vi "New Client Handle.vi"(8 "error in (no error)":errorcluster, 11 "REST Client in":refnum<class "REST Client.lvclass">) -> (0 "error out":errorcluster, 2 "Client Handle":refnum<class "Abstract HTTP Client.lvclass">, 3 "REST Client out":refnum<class "REST Client.lvclass">)   [LabVIEW 2020, in "REST Client.lvlib" / "REST Client.lvclass"]
uses:
  REST Client.lvclass
  <vilib>/VIPM Community/HTTP Client Plugin - Base/Classes/Abstract HTTP Client/Abstract HTTP Client.lvclass
  REST Client.lvclass/REST Client.ctl
  <vilib>/VIPM Community/HTTP Client Plugin - Base/Classes/LabVIEW HTTP Client/LabVIEW HTTP Client.lvclass
  C:/Program Files/National Instruments/LabVIEW 2025/vi.lib/VIPM Community/HTTP Client Plugin - Base/Classes/LabVIEW HTTP Client/LabVIEW HTTP Client.lvclass
  C:/Program Files/National Instruments/LabVIEW 2025/vi.lib/VIPM Community/HTTP Client Plugin - Base/Classes/Abstract HTTP Client/Abstract HTTP Client.lvclass
panel:
  in  "http-client-type":refnum<class "Abstract HTTP Client.lvclass">
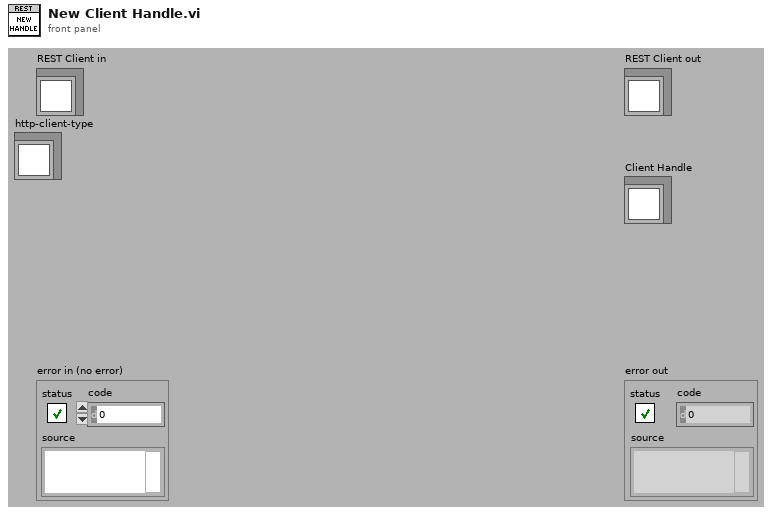
[diagram p1: front panel]
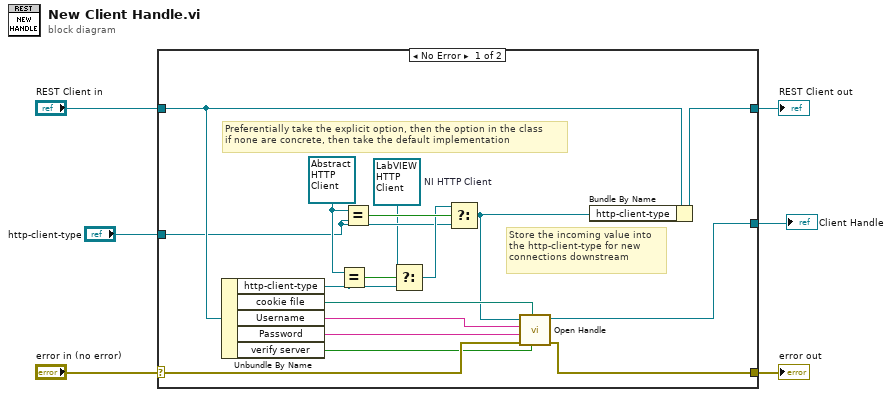
[diagram p0: block diagram]
diagram:
  n1 = case shown="No Error" "error in (no error)" {
    selector: "error in (no error)" -> [w23 w25]
    tunnel: [w17 w25] -> w5
    tunnel: [w9 w24] -> w3
    tunnel: "REST Client in" -> [w22 w24]
    tunnel: "http-client-type" -> [w11 _]
    tunnel: [w10 _] -> w1
    frame No Error {
      w7 = refnum<class "LabVIEW HTTP Client.lvclass"> refnum  # NI HTTP Client
      w15 = refnum<class "Abstract HTTP Client.lvclass"> refnum ("x")
      # "Store the incoming value into\nthe http-client-type for new\nconnections downstream"
      # "Preferentially take the explicit option, then the option in the class\nif none are concrete, then take the default implementation"
      n2 = Unbundle By Name(w22) -> ("http-client-type"=w13:refnum<class "Abstract HTTP Client.lvclass">, "cookie file"=w19:path, "Username"=w21:string, "Password"=w20:string, "verify server"=w18:bool)
      n3 = Equal?(x=w15, y=w13) -> (x = y?=w14:bool)
      n4 = Equal?(x=w15, y=w11) -> (x = y?=w16:bool)
      n5 = Select(t=w7, s=w14, f=w13) -> (s? t:f=w12:refnum<class "Abstract HTTP Client.lvclass">)
      n6 = Select(t=w12, s=w16, f=w11) -> (s? t:f=w8:refnum<class "Abstract HTTP Client.lvclass">)
      n7 = call-dynamic "Open Handle.vi"("verify server(true)"=w18, "cookie file"=w19, "error in (no error)"=w23, "password"=w20, "username"=w21, "HTTP Client Abstract in"=w8) -> ("error out"=w17:errorcluster, "HTTP Client Abstract out"=w10:refnum<class "Abstract HTTP Client.lvclass">)  [unwired: 4 in]
      n8 = Bundle By Name(cluster=w22, "http-client-type"=w8) -> (w9:refnum<class "REST Client.lvclass">)
    }
    frame Error {
    }
  }
  "error out" <- w5
  "REST Client out" <- w3
  "Client Handle" <- w1
